vi "Get__slk_mt.vi"(8 "error in (no error)":errorcluster, 11 "digital u32 in":refnum<class "Digital U32__slk_mt.lvclass">) -> (0 "error out":errorcluster, 3 "digital u32 out":refnum<class "Digital U32__slk_mt.lvclass">, 5 "value":string[](array[string]))   [LabVIEW 2013, in "Lazyboots Menu Tool.lvlib" / "Digital U32__slk_mt.lvclass"]
doc: "Gets the value from the control on GUI.\n\n<b>Value:</b>\n[Section, Key, Value]"
uses:
  Digital U32__slk_mt.lvclass
panel:
  # "Get__slk_mt.vi\nGets the values from the control on GUI.\n\nNOTICE -- YOU MUST LEAVE THIS NOTICE IN PLACE.\n\nCopyright (c) 2011, LIANG LIU Shawn.Liu.cn@gmail.com\nAll rights reserved.\n\nRedistribution and use in source and binary forms, with or without modification, are permitted provided that the following conditions are met:\n-Redistributions of source code must retain the above copyright notice, this list of conditions and the following disclaimer.\n-Redistributions in binary form must reproduce the above copyright notice, this list of conditions and the following disclaimer in the documentation and/or other materials provided with the distribution.\n-Neither the name of the eLp nor the names of its contributors may be used to endorse or promote products derived from this software without specific prior written permission.\n\nTHIS SOFTWARE IS PROVIDED BY THE COPYRIGHT HOLDERS AND CONTRIBUTORS \"AS IS\" AND ANY EXPRESS OR IMPLIED WARRANTIES, INCLUDING, BUT NOT LIMITED TO, THE IMPLIED WARRANTIES OF MERCHANTABILITY AND FITNESS FOR A PARTICULAR PURPOSE ARE DISCLAIMED. IN NO EVENT SHALL THE COPYRIGHT HOLDER OR CONTRIBUTORS BE LIABLE FOR ANY DIRECT, INDIRECT, INCIDENTAL, SPECIAL, EXEMPLARY, OR CONSEQUENTIAL DAMAGES (INCLUDING, BUT NOT LIMITED TO, PROCUREMENT OF SUBSTITUTE GOODS OR SERVICES; LOSS OF USE, DATA, OR PROFITS; OR BUSINESS INTERRUPTION) HOWEVER CAUSED AND ON ANY THEORY OF LIABILITY, WHETHER IN CONTRACT, STRICT LIABILITY, OR TORT (INCLUDING NEGLIGENCE OR OTHERWISE) ARISING IN ANY WAY OUT OF THE USE OF THIS SOFTWARE, EVEN IF ADVISED OF THE POSSIBILITY OF SUCH DAMAGE."
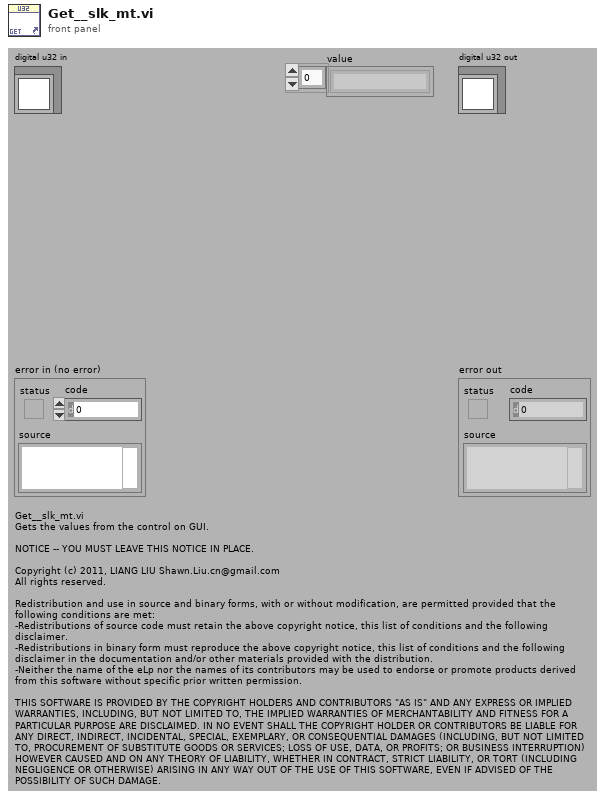
[diagram p1: front panel]
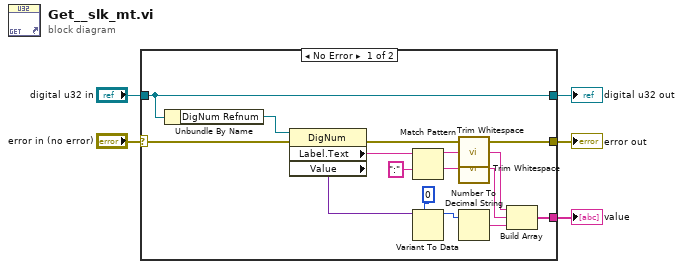
[diagram p0: block diagram]
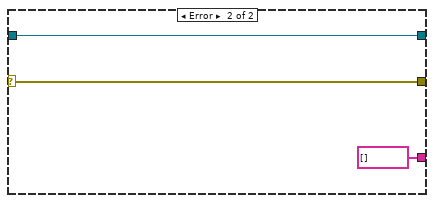
[diagram p2: hidden frame]
diagram:
  n1 = case shown="No Error" "error in (no error)" {
    selector: "error in (no error)" -> [w7 w23]
    tunnel: [w9 w23] -> w5
    tunnel: [w8 string[] []] -> w4
    tunnel: "digital u32 in" -> [w6 w21]
    tunnel: [w6 w21] -> w1
    frame No Error {
      n2 = Unbundle By Name(w6) -> ("DigNum Refnum"=w20:refnum<vi>)
      n3 = property class="DigNum"(reference=w20, error in=w7) -> (error out=w9:errorcluster, "Label.Text"=w19:string, "Value"=w15:variant)  [unwired: 1 out]
      n4 = Match Pattern(string=w19, regular expression=":") -> (before substring=w17:string, after substring=w16:string)  [unwired: 1 in, 2 out]
      n5 = Variant To Data(type=u32 0, Variant=w15) -> (data=w13:u32)  [unwired: 1 in, 1 out]
      n6 = call <vilib>:"Trim Whitespace.vi"("string"=w17) -> ("trimmed string"=w12:string)  [unwired: 1 in]
      n7 = call <vilib>:"Trim Whitespace.vi"("string"=w16) -> ("trimmed string"=w11:string)  [unwired: 1 in]
      n8 = Number To Decimal String(number=w13) -> (decimal integer string=w10:string)  [unwired: 1 in]
      n9 = Build Array(w12, w11, w10) -> (w8:string[])
    }
    frame Error {
    }
  }
  "error out" <- w5
  "digital u32 out" <- w1
  "value" <- w4
